vi "Read Macro LUT (Name-_Macro).vi"(11 "Motions in":refnum<class "Motions.lvclass">) -> (2 "Macro LUT (Name->Macro)":variant, 3 "Motions out":refnum<class "Motions.lvclass">)   [LabVIEW 2016, in "Hardware.lvlib" / "Motions.lvlib" / "Motions.lvclass"]
uses:
  <userlib>/Common Components/Hardware/Abstract System/Motions/Motions/Motions.lvclass
  <userlib>/Common Components/Hardware/Abstract System/Motions/Motions/Motions.lvclass/Motions.ctl
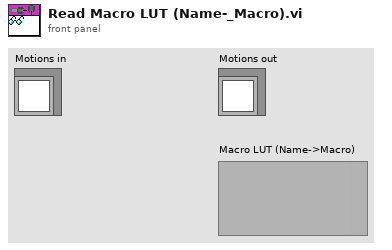
[diagram p1: front panel]
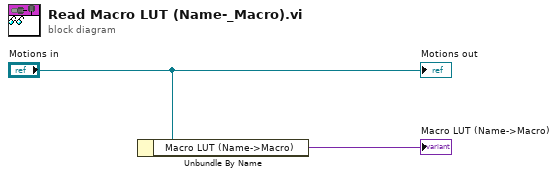
[diagram p0: block diagram]
diagram:
  n1 = Unbundle By Name("Motions in") -> ("Macro LUT (Name->Macro)"=→"Macro LUT (Name->Macro)":variant)
  "Motions out" <- "Motions in"
